vi "SV Get Software Trigger Parameters.vi"(0 "scaled signals [EU] in":waveform(dbl)[](array[waveform]), 11 "error in (no error)":errorcluster) -> (3 "trigger channel found":bool, 4 "scaled signals [EU] out":waveform(dbl)[](array[waveform]), 6 "level trigger configuration":T1={"level"=0.0, "slope"=1, "hysteresis"=0.0} {"hysteresis" format="%.2p"; "slope" items=["Falling Edge", "Rising Edge"]; "level" format="%.2p"}, 8 "trigger index":i32, 10 "trigger channel name":string, 13 "data timestamp":timestamp, 14 "pretrigger samples":i32, 15 "error out":errorcluster)   [LabVIEW 2017]
uses:
  <vilib>/addons/_NISVFA/_Shared subVIs/Controls/SV Channel Properties.ctl
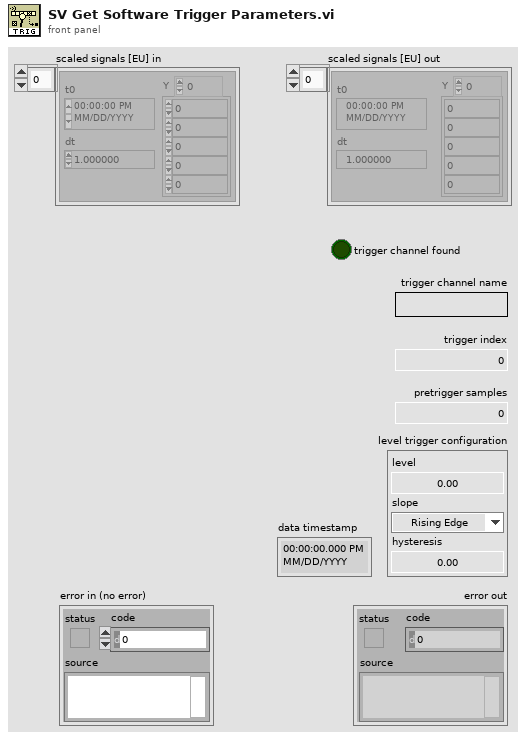
[diagram p1: front panel]
types:
  T1 = cluster{"level":dbl, "slope":u16, "hysteresis":dbl}
  T2 = typedef "SV Channel Properties.ctl" = u16
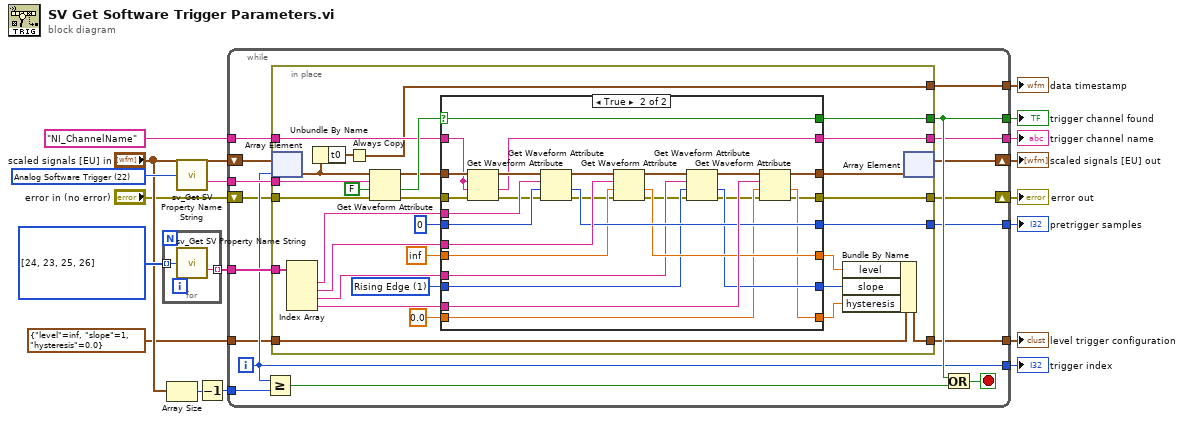
[diagram p0: block diagram]
diagram:
  w10 = T2 22 items=["Engineering units", "Custom unit label", "Weighting filter", "Pregain", "Octave standard", "Octave bandwidth", "Octave low band", "Octave high band", "Spectrum skewed", "Samples / revolution", "Order", "Tachometer", "Pulses Per Revolution", "Rotation Direction", "Probe Angle", "Pair", "Channel Alias", "Tachometer Threshold", "Tachometer Slope", "Max Order", "Sensor Location", "Sensor Orientation", "Analog Software Trigger", "Trigger Level", "Pretrigger Samples", "Trigger Slope", "Trigger Hysteresis"] ("SV property")
  w9 = T2[] [24, 23, 25, 26] items=["Engineering units", "Custom unit label", "Weighting filter", "Pregain", "Octave standard", "Octave bandwidth", "Octave low band", "Octave high band", "Spectrum skewed", "Samples / revolution", "Order", "Tachometer", "Pulses Per Revolution", "Rotation Direction", "Probe Angle", "Pair", "Channel Alias", "Tachometer Threshold", "Tachometer Slope", "Max Order", "Sensor Location", "Sensor Orientation", "Analog Software Trigger", "Trigger Level", "Pretrigger Samples", "Trigger Slope", "Trigger Hysteresis"]
  n1 = for {
    tunnel: w9 -> [w20] mode=indexing
    tunnel: [w19] -> w12 mode=indexing
    n2 = call <vilib>:"sv_Get SV Property Name String.vi"("property"=w20) -> ("WDT attribute name"=w19:string)  [unwired: 13 in, 1 out]
  }
  n3 = Array Size(array="scaled signals [EU] in") -> (size(s)=w6:i32)
  n4 = call <vilib>:"sv_Get SV Property Name String.vi"("property"=w10) -> ("WDT attribute name"=w11:string)  [unwired: 13 in, 1 out]
  n5 = Decrement(x=w6) -> (x-1=w7:i32)
  n6 = while {
    tunnel: w7 -> [w37]
    tunnel: [w34] -> w15
    tunnel: [w27] -> w17
    shift-right: [w31] -> w16
    shift-left: "scaled signals [EU] in" -> [w32]
    tunnel: w11 -> [w33]
    tunnel: w12 -> [w30]
    tunnel: [w28] -> w14
    tunnel: [w26] -> w18
    tunnel: "NI_ChannelName" ("name") -> [w25]
    shift-right: [w23] -> w3
    shift-left: "error in (no error)" -> [w24]
    tunnel: T1 {"level"=inf, "slope"=1, "hysteresis"=0.0} ("level trigger configuration") -> [w22]
    tunnel: [w29] -> w13
    tunnel: [w21] -> w1
    i -> [w27]
    stop <- w36 stop-if-true
    n7 = Greater Or Equal?(x=w27, y=w37) -> (x >= y?=w35:bool)
    n8 = in-place {
      in-place-border: [w56] -> w34
      in-place-border: w33 -> [w65]
      in-place-border: w30 -> [w58]
      in-place-border: [w48] -> w29
      in-place-border: [w47] -> w28
      in-place-border: [w46] -> w26
      in-place-border: w25 -> [w45]
      in-place-border: w24 -> [w44]
      in-place-border: [w42] -> w23
      in-place-border: w22 -> [w41]
      in-place-border: [w38] -> w21
      w51 = u16 1 items=["Falling Edge", "Rising Edge"] ("slope")
      n9 = in-place-array #1(w32, w27) -> (w40:waveform(dbl))
      n10 = Index Array(array=w58) -> (element #1=w59:string, element #2=w60:string, element #3=w61:string, element #4=w49:string)  [unwired: 4 in]
      n11 = Unbundle By Name(w40) -> ("t0"=w39:timestamp)
      n12 = Always Copy(1:w39) -> (0:w38:timestamp)
      n13 = Get Waveform Attribute(4:w44, 5:FALSE, 6:w65, 7:w40) -> (0:w43:errorcluster, 1:w57:bool, 3:w54:waveform(dbl))  [unwired: 1 out]
      n14 = case shown="True" w57 {
        selector: w57 -> [w68 w84]
        tunnel: w59 -> [_ w100]
        tunnel: w60 -> [_ w99]
        tunnel: w61 -> [_ w87]
        tunnel: w49 -> [_ w95]
        tunnel: [w73 w94] -> w47
        tunnel: [w72 w93] -> w62
        tunnel: [w71 w92] -> w63
        tunnel: [w70 w91] -> w64
        tunnel: 0 -> [w73 w90]
        tunnel: inf -> [w72 w89]
        tunnel: w51 -> [w71 w88]
        tunnel: 0.0 -> [w70 w86]
        tunnel: [w68 w84] -> w56
        tunnel: [w69 w85] -> w55
        tunnel: w54 -> [w69 w82]
        tunnel: w45 -> [_ w81]
        tunnel: [_ w80] -> w46
        tunnel: w43 -> [w67 w79]
        tunnel: [w67 w74] -> w42
        frame False {
        }
        frame True {
          n15 = Get Waveform Attribute(4:w79, 5:w81, 6:w81, 7:w82) -> (0:w78:errorcluster, 1:w80:string, 3:w83:waveform(dbl))  [unwired: 1 out]
          n16 = Get Waveform Attribute(4:w78, 5:w90, 6:w100, 7:w83) -> (0:w77:errorcluster, 1:w94:i32, 3:w98:waveform(dbl))  [unwired: 1 out]
          n17 = Get Waveform Attribute(4:w77, 5:w89, 6:w99, 7:w98) -> (0:w76:errorcluster, 1:w93:dbl, 3:w97:waveform(dbl))  [unwired: 1 out]
          n18 = Get Waveform Attribute(4:w76, 5:w88, 6:w87, 7:w97) -> (0:w75:errorcluster, 1:w92:u16, 3:w96:waveform(dbl))  [unwired: 1 out]
          n19 = Get Waveform Attribute(4:w75, 5:w86, 6:w95, 7:w96) -> (0:w74:errorcluster, 1:w91:dbl, 3:w85:waveform(dbl))  [unwired: 1 out]
        }
      }
      n20 = Bundle By Name(cluster=w41, "level"=w62, "slope"=w63, "hysteresis"=w64) -> (w48:T1)
      n21 = in-place-array #1(w55) -> (w31:waveform(dbl)[])  [unwired: 1 out]
    }
    n22 = Or(x=w34, y=w35) -> (x .or. y?=w36:bool)
  }
  "trigger channel name" <- w18
  "trigger index" <- w17
  "scaled signals [EU] out" <- w16
  "trigger channel found" <- w15
  "pretrigger samples" <- w14
  "level trigger configuration" <- w13
  "error out" <- w3
  "data timestamp" <- w1
